vi "CRYPIC Replace Frame Title.vi"(9 "sNewTitle":string, 10 "tFrame":T2) -> (2 "tFrame_Out":T2)   [LabVIEW 2013]
uses:
  <vilib>/Utility/miscctls.llb/LVRectTypeDef.ctl
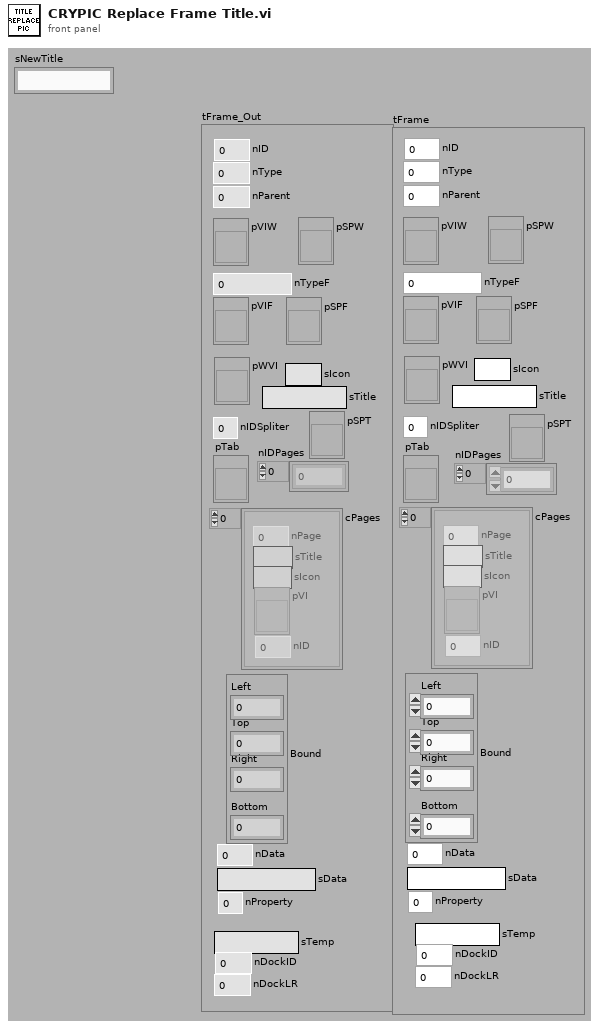
[diagram p1: front panel]
types:
  T1 = typedef "LVRectTypeDef.ctl" = cluster{"Left":i16, "Top":i16, "Right":i16, "Bottom":i16}
  T2 = cluster{"nType":i32, "nParent":i32, "pVIW":refnum<vi>, "pSPW":refnum<vi>, "nTypeF":i32, "pVIF":refnum<vi>, "pSPF":refnum<vi>, "nIDSpliter":i32, "nProperty":i32, "Bound":T1, "nID":i32, "nData":i32, "sData":string, "pWVI":refnum<vi>, "sTitle":string, "cPages":cluster{"nPage":i32, "sTitle":string, "sIcon":string, "pVI":refnum<vi>, "nID":i32}[], "pTab":refnum<vi>, "nIDPages":i32[], "pSPT":refnum<vi>, "sTemp":string, "nDockID":i32, "nDockLR":i32, "sIcon":string}
  T3 = cluster{"nPage":i32, "sTitle":string, "sIcon":string, "pVI":refnum<vi>, "nID":i32}[]
  T4 = cluster{"nPage":i32, "sTitle":string, "sIcon":string, "pVI":refnum<vi>, "nID":i32}
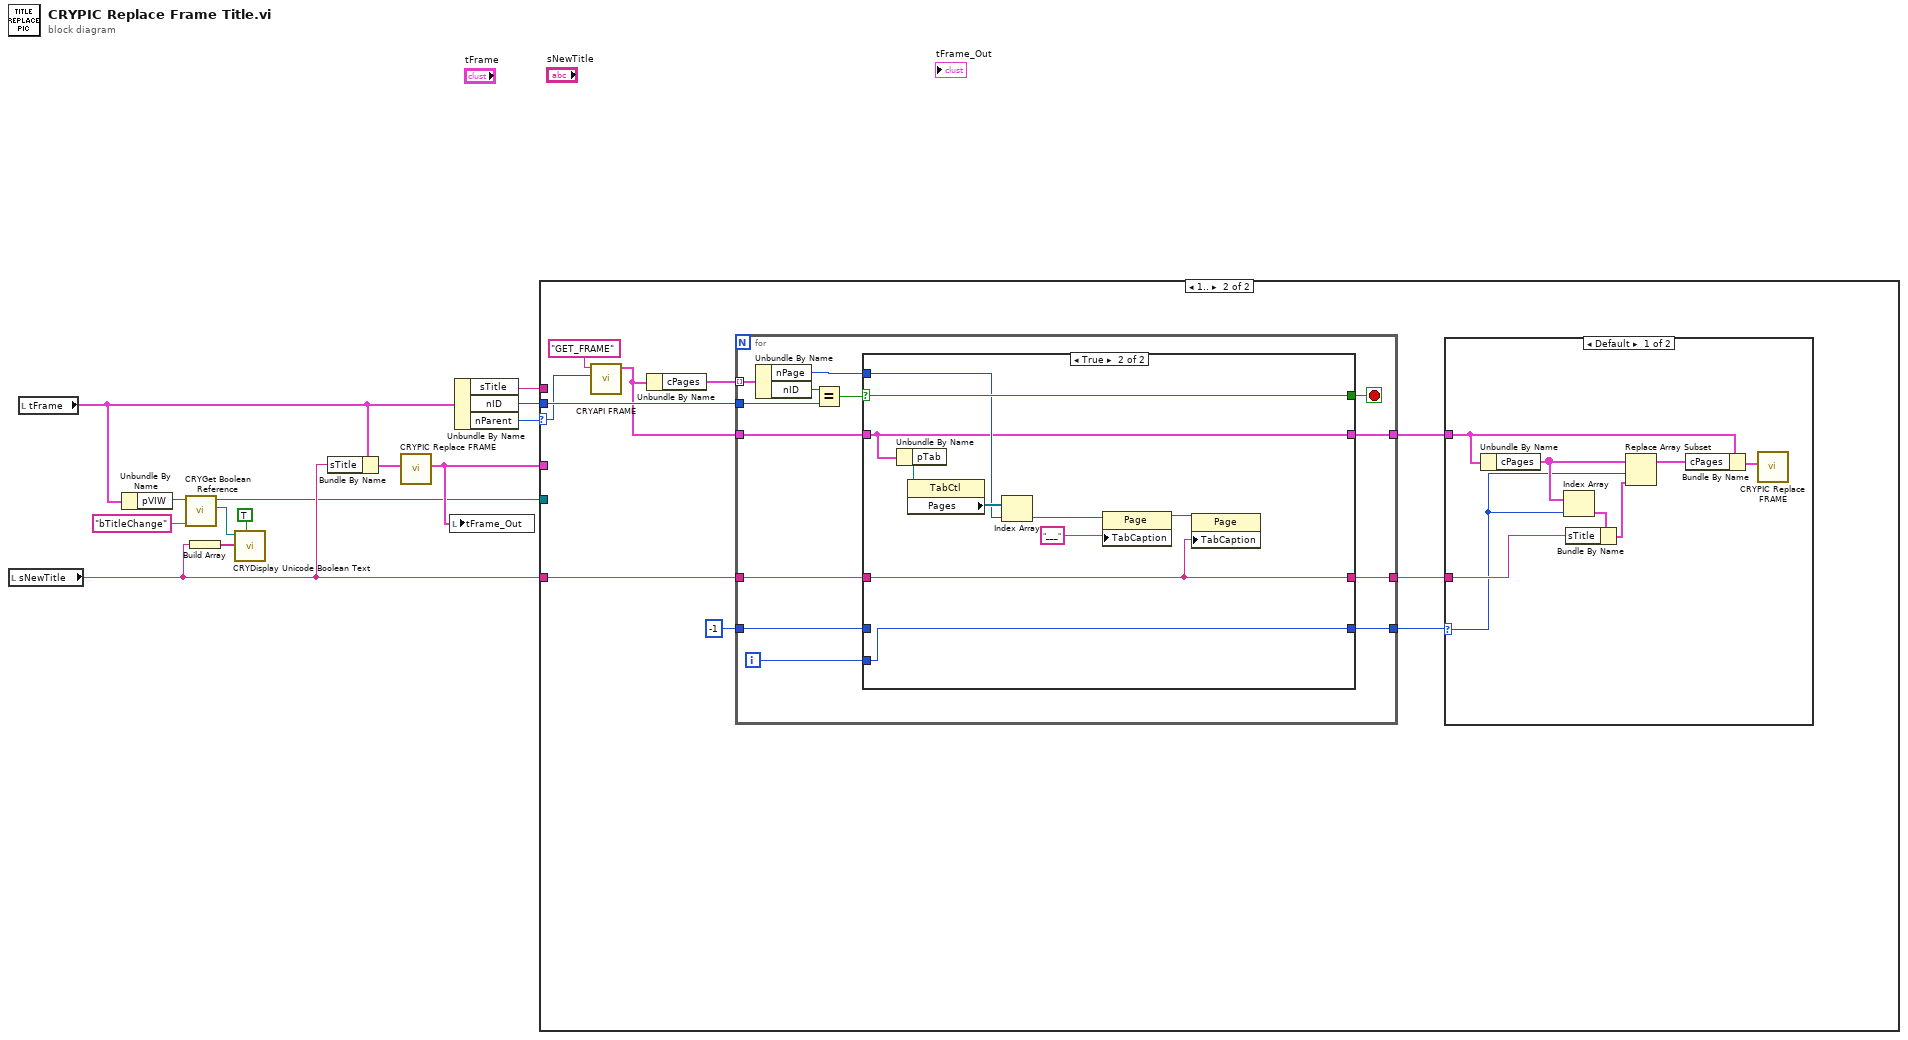
[diagram p0: block diagram]
diagram:
  n1 = local read "sNewTitle"() -> (w4:string)
  n2 = local read "tFrame"() -> (w9:T2)
  n3 = Unbundle By Name(w9) -> ("pVIW"=w3:refnum<vi>)
  n4 = call "CRYGet Boolean Reference.vi"("Label Name"="bTitleChange" ("Control Name"), "VI Refnum"=w3) -> ("Boolean Ref"=w5:refnum<vi>, "VI Refnum Out"=w2:refnum<vi>)  [unwired: 7 in, 1 out]
  n5 = Build Array(w4) -> (w7:string[])
  n6 = call "CRYDisplay Unicode Boolean Text.vi"("Interpret as Unicode (T)"=TRUE, "Boolean Texts [4]"=w7, "Boolean Reference"=w5) -> ()  [unwired: 5 in, 2 out]
  n7 = Bundle By Name(cluster=w9, "sTitle"=w4) -> (w10:T2)
  n8 = call "CRYPIC Replace FRAME.vi"("tFrame"=w10) -> ("tFrame_Out"=w8:T2)  [unwired: 10 in]
  n9 = local write "tFrame_Out"(w8) -> ()
  n10 = Unbundle By Name(w9) -> ("sTitle"=w11:string, "nID"=w12:i32, "nParent"=w13:i32)
  n11 = case shown="1.." w13 {
    selector: w13 -> [_ w21]
    tunnel: w12 -> [_ w23]
    tunnel: w11 -> [_ _]
    tunnel: w4 -> [_ w18]
    tunnel: w8 -> [_ _]
    tunnel: w2 -> [_ _]
    frame ..0, Default {
    }
    frame 1.. {
      n12 = call "CRYAPI FRAME.vi"("nData"=w21, "sAction"="GET_FRAME") -> ("tFrame_Out"=w19:T2)  [unwired: 4 in, 5 out]
      n13 = Unbundle By Name(w19) -> ("cPages"=w20:T3)
      n14 = for {
        tunnel: w20 -> [w44] mode=indexing
        tunnel: w23 -> [w42]
        tunnel: w19 -> [w40]
        tunnel: w18 -> [w37]
        tunnel: -1 -> [w36]
        tunnel: [w35] -> w16
        tunnel: [w33] -> w14
        tunnel: [w32] -> w15
        i -> [w34]
        stop <- w38 stop-if-true
        n15 = Unbundle By Name(w44) -> ("nPage"=w39:i32, "nID"=w43:i32)
        n16 = Equal?(x=w43, y=w42) -> (x = y?=w41:bool)
        n17 = case shown="True" w41 {
          selector: w41 -> [w48 w58]
          tunnel: w40 -> [w45 w54]
          tunnel: w39 -> [_ w56]
          tunnel: [w48 w58] -> w38
          tunnel: w37 -> [w46 w52]
          tunnel: w36 -> [w47 _]
          tunnel: [w47 w55] -> w35
          tunnel: w34 -> [_ w55]
          tunnel: [w46 w52] -> w33
          tunnel: [w45 w54] -> w32
          frame False {
          }
          frame True {
            n18 = Unbundle By Name(w54) -> ("pTab"=w53:refnum<vi>)
            n19 = property class="TabCtl"(reference=w53) -> ("Pages"=w57:refnum<vi>[])  [unwired: 1 in, 2 out]
            n20 = Index Array(array=w57, index=w56) -> (element=w51:refnum<vi>)
            n21 = property class="Page"(reference=w51, "TabCaption"="___" ("string")) -> (reference out=w50:refnum<vi>)  [unwired: 1 in, 1 out]
            n22 = property class="Page"(reference=w50, "TabCaption"=w52) -> ()  [unwired: 1 in, 2 out]
          }
        }
      }
      n23 = case shown="Default" w16 {
        selector: w16 -> [w27 _]
        tunnel: w15 -> [w26 _]
        tunnel: w14 -> [w30 _]
        frame Default {
          n24 = Unbundle By Name(w26) -> ("cPages"=w29:T3)
          n25 = Index Array(array=w29, index=w27) -> (element=w31:T4)
          n26 = Bundle By Name(cluster=w31, "sTitle"=w30) -> (w28:T4)
          n27 = Replace Array Subset(array=w29, new element=w28, index=w27) -> (w25:T3)
          n28 = Bundle By Name(cluster=w26, "cPages"=w25) -> (w24:T2)
          n29 = call "CRYPIC Replace FRAME.vi"("tFrame"=w24) -> ()  [unwired: 10 in, 1 out]
        }
        frame -1 {
        }
      }
    }
  }
